vi "User32dllAPI.CloseWindow.vi"(8 "error in (no error)":errorcluster, 11 "hWnd":i32) -> (0 "error out":errorcluster, 3 "hWnd out":i32)   [LabVIEW 2010]
uses:
  user32.dll
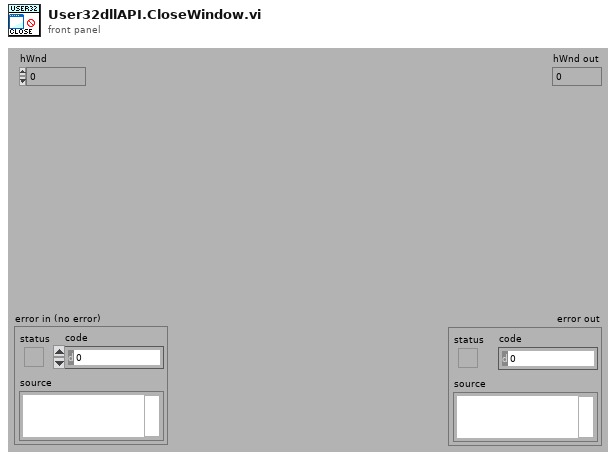
[diagram p1: front panel]
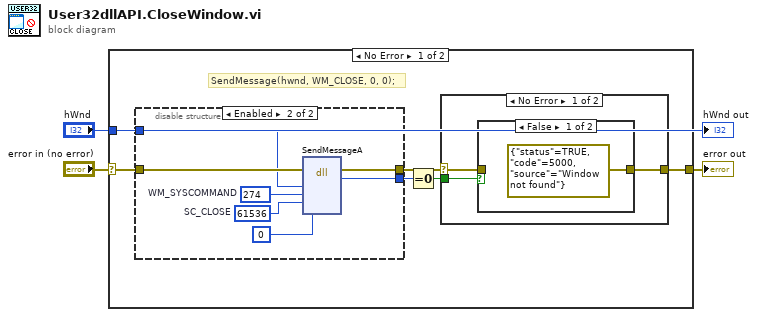
[diagram p0: block diagram]
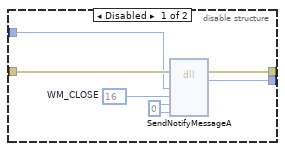
[diagram p2: hidden frame]
diagram:
  n1 = case shown="No Error" "error in (no error)" {
    selector: "error in (no error)" -> [w8 w29]
    tunnel: [w6 w29] -> w2
    tunnel: "hWnd" -> [w5 _]
    frame No Error {
      # "SendMessage(hwnd, WM_CLOSE, 0, 0);"
      n2 = disable-structure shown="Enabled" {
        disable-tunnel: w8 -> [w15 w17]
        disable-tunnel: [w14 w19] -> w7
        disable-tunnel: w5 -> [w13 w16]
        disable-tunnel: [w12 w18] -> w4
        frame Disabled {
          w10 = 0
          w11 = u32 16  # WM_CLOSE
          n3 = dll-call lib="USER32.DLL" fn="SendNotifyMessageA" label="SendNotifyMessage"(error in=w15, "hWnd"=w13, "Msg"=w11, "wParam"=w10, "lParam"=w10) -> (error out=w14:errorcluster, "result"=w12:i32)  [unwired: 6 in, 1 out]
        }
        frame Enabled {
          w21 = 61536  # SC_CLOSE
          w22 = u32 274  # WM_SYSCOMMAND
          n4 = dll-call lib="USER32.DLL" fn="SendMessageA" label="SendMessage"(error in=w17, "hWnd"=w16, "Msg"=w22, "wParam"=w21, "lParam"=0) -> (error out=w19:errorcluster, "result"=w18:i32)  [unwired: 6 in, 1 out]
        }
      }
      n5 = Equal To 0?(x=w4) -> (x = 0?=w9:bool)
      n6 = case shown="No Error" w7 {
        selector: w7 -> [w23 w28]
        tunnel: w9 -> [w25 _]
        tunnel: [w24 w28] -> w6
        frame No Error {
          n7 = case shown="False" w25 {
            tunnel: [errorcluster {"status"=TRUE, "code"=5000, "source"="Window not found"} ("error out") w27] -> w24
            tunnel: w23 -> [_ w27]
            frame False {
            }
            frame True {
            }
          }
        }
        frame Error {
        }
      }
    }
    frame Error {
    }
  }
  "error out" <- w2
  "hWnd out" <- "hWnd"
